vi "两边沿间隔_连续.vi"() -> ()   [LabVIEW 2013]
uses:
  <userlib>/ArtDAQ/_SubVI/ArtDAQ_CreateCITwoEdgeSepChan.vi
  <userlib>/ArtDAQ/_SubVI/ArtDAQ_CfgImplicitTiming.vi
  <userlib>/ArtDAQ/_SubVI/ArtDAQ_Read Counter DBL NSamp.vi
panel:
  in  "第二个边沿":i32(ring)=10280 items=["上升"=10280, "下降"=10171]
  in  "第一个边沿":i32(ring)=10280 items=["上升"=10280, "下降"=10171]
  in  "每通道点数":i32=100
  in  "Stop":bool
  out "数据":dbl[](array[numeric])
  in  "计数器":string="Dev1/ctr0"
  in  "最小值":dbl=1e-06 format="%0.6f"
  in  "最大值":dbl=10.0 format="%0.6f"
  out "错误输出":errorcluster
  # "通道属性"
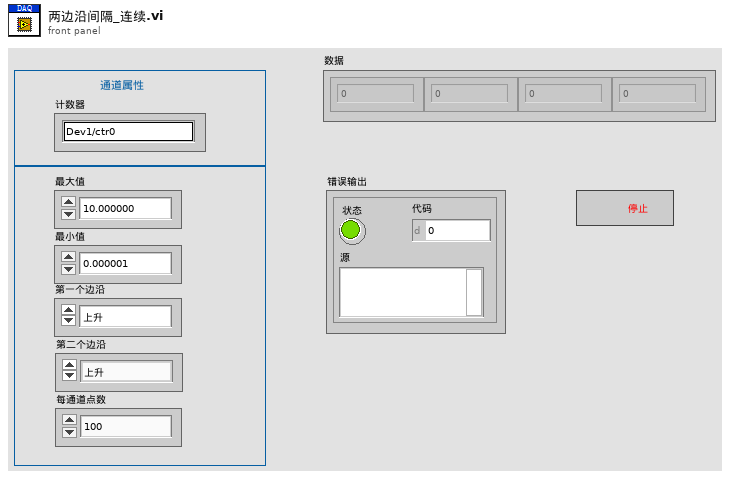
[diagram p1: front panel]
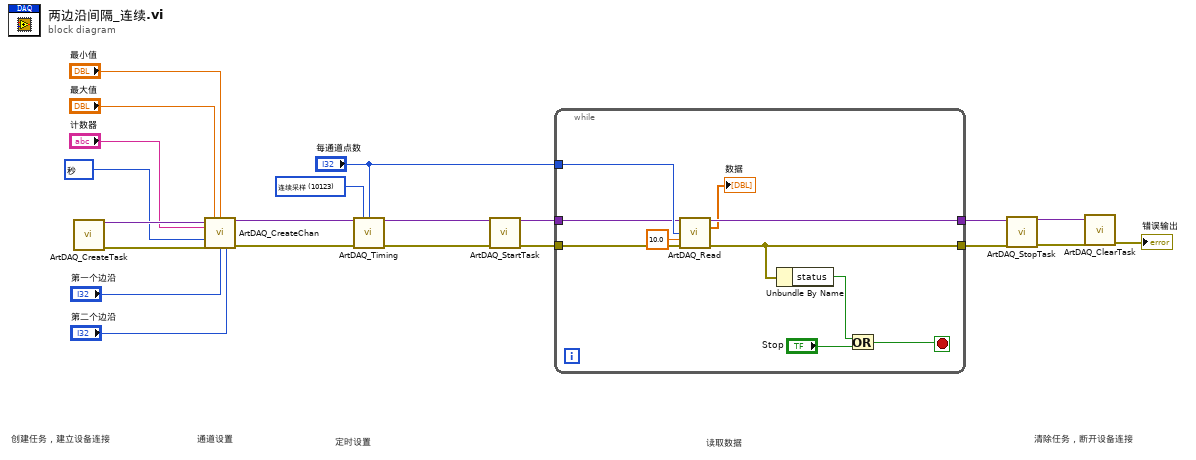
[diagram p0: block diagram]
diagram:
  w5 = 10364 items=["秒"=10364, "时钟滴答"=10304, "来自自定义换算"=10065] ("Units")
  w9 = 10123 items=["有限点采样"=10178, "连续采样"=10123] ("SampleMode")
  # "清除任务，断开设备连接"
  # "读取数据"
  # "定时设置"
  # "通道设置"
  # "创建任务，建立设备连接"
  n1 = call <userlib>:"ArtDAQ_CreateTask.vi"() -> ("任务句柄"=w21:variant, "错误输出"=w20:errorcluster)  [unwired: 14 in]
  n2 = call-poly <userlib>:"ArtDAQ_CreateChan.vi"("任务句柄"=w21, "最大值"="最大值", "最小值"="最小值", "计数器"="计数器", "单位"=w5, "错误输入"=w20, "第一个边沿"="第一个边沿", "第二个边沿"="第二个边沿") -> ("任务句柄"=w11:variant, "错误输出"=w10:errorcluster)  [unwired: 6 in]
  n3 = call-poly <userlib>:"ArtDAQ_Timing.vi"("任务句柄"=w11, "采样模式"=w9, "每通道采样数"="每通道点数", "错误输入"=w10) -> ("任务句柄"=w7:variant, "错误输出"=w6:errorcluster)  [unwired: 10 in]
  n4 = call <userlib>:"ArtDAQ_StartTask.vi"("任务句柄"=w7, "错误输入"=w6) -> ("任务句柄"=w2:variant, "错误输出"=w1:errorcluster)  [unwired: 12 in]
  n5 = while {
    tunnel: [w31] -> w18
    tunnel: [w30] -> w16
    tunnel: "每通道点数" -> [w29]
    tunnel: w2 -> [w24]
    tunnel: w1 -> [w23]
    stop <- w22 stop-if-true
    n6 = call-poly <userlib>:"ArtDAQ_Read.vi"("任务句柄"=w24, "每通道采样数"=w29, "超时s"=10.0 ("Timeout"), "错误输入"=w23) -> ("任务句柄"=w31:variant, "数据"=→"数据":dbl[], "错误输出"=w30:errorcluster)  [unwired: 8 in, 1 out]
    n7 = Unbundle By Name(w30) -> ("status"=w26:bool)
    n8 = Or(x=w26, y="Stop") -> (x .or. y?=w22:bool)
  }
  n9 = call <userlib>:"ArtDAQ_StopTask.vi"("任务句柄"=w18, "错误输入"=w16) -> ("任务句柄"=w17:variant, "错误输出"=w15:errorcluster)  [unwired: 12 in]
  n10 = call <userlib>:"ArtDAQ_ClearTask.vi"("任务句柄"=w17, "错误输入"=w15) -> ("错误输出"=→"错误输出":errorcluster)  [unwired: 13 in]
